vi "genIOL_realtime_traj.vi"() -> ()   [LabVIEW 2016]
panel:
  out "1-D Array of Real 2":dbl[](array[numeric])
  out "1-D Array of Real":dbl[](array[numeric])
  in  "Bscan path":path=path "D:/IRISSoft LV2016 beta/Host Demo/ThorlabsData/Incision Bscan/test.png"
  in  "size_xyz":dbl[](array[numeric])=[400.0, 400.0, 1024.0, 1.0]
  in  "size_xyz_mm":dbl[](array[numeric])=[16.0, 16.0, 9.4, 1.0]
  in  "incision row range":dbl=0.09
  in  "Incision point":dbl[](array[numeric])=[5.0, 9.897598828696928, 1.731822640236092]
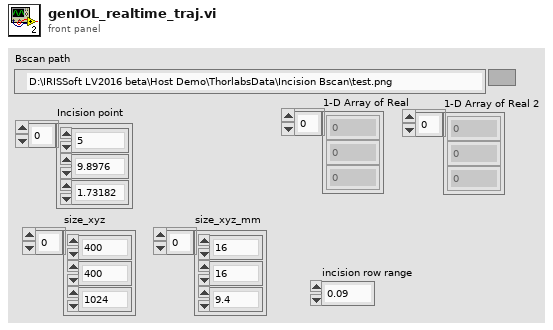
[diagram p1: front panel]
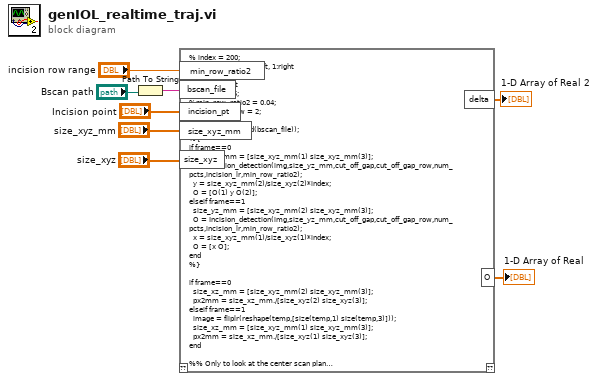
[diagram p0: block diagram]
diagram:
  n1 = Path To String(path="Bscan path") -> (string=w4:string)
  n2 = script code="% index = 200;\nincision_lr = 0; % 0:left, 1:right\ncut_off_gap = 3.5;\n% 0 < init_pct\nnum_pcts = 5;\n%min_row_ratio2 = 0.04;\ncut_off_gap_row = 2;\n\nimg = fliplr(imread(bscan_file));\n%{\nif frame==0\n  size_yz_mm = [size_xyz_mm(1) size_xyz_mm(3)];\n  O = Incision_detection(img,size_yz_mm,cut_off_gap,cut_off_gap_row,num_pcts,incision_lr,min_row_ratio2);\n  y = size_xyz_mm(2)/size_xyz(2)*index;\n  O = [O(1) y O(2)];\nelseif frame==1\n  size_yz_mm = [size_xyz_mm(2) size_xyz_mm(3)];\n  O = Incision_detection(img,size_yz_mm,cut_off_gap,cut_off_gap_row,num_pcts,incision_lr,min_row_ratio2);\n  x = size_xyz_mm(1)/size_xyz(1)*index;\n  O = [x O];\nend\n%}\n\nif frame==0\n  size_xz_mm = [size_xyz_mm(2) size_xyz_mm(3)];\n  px2mm = size_xz_mm./[size_xyz(2) size_xyz(3)]; \nelseif frame==1\n  image = fliplr(reshape(temp,[size(temp,1) size(temp,3)]));\n  size_xz_mm = [size_xyz_mm(1) size_xyz_mm(3)];\n  px2mm = size_xz_mm./[size_xyz(1) size_xyz(3)]; \nend\n\n%% Only to look at the center scan plan\nfigure(2); clf; \nimshow(img); hold on;\n    \n% Collect two user clicks of Injection location \n[input1, Zinput1] = ginput(1);\nplot(input1, Zinput1, 'rx', 'MarkerSize', 20, 'LineWidth', 3); \n[input2, Zinput2] = ginput(1); % Collect two user clicks \nplot(input2, Zinput2, 'rx', 'MarkerSize', 20, 'LineWidth', 3); \nif frame==1\n  Yinput1 = size_xyz(2) - input1; \n  Yinput2 = size_xyz(2) - input2;\nelseif frame==0\n  Yinput1 = size_xyz(1) - input1; \n  Yinput2 = size_xyz(1) - input2;\nend\n\nINJECTloc_px = [Yinput1, Zinput1; ... \n        Yinput2, Zinput2]; % [px] \nINJECTloc_px_mid=[(INJECTloc_px(1,1)+INJECTloc_px(2,1))/2,(INJECTloc_px(1,2)+INJECTloc_px(2,2))/2];\nclose(2); % close figure\n    \n% Convert these two locations from pixels to {OCT} frame  \nxloc_OCT = index/400*size_xz_mm(1); % B-scan is halfway through the image\nINJECTloc_OCT = [xloc_OCT*ones(1,1), INJECTloc_px_mid(1,1)*px2mm(1),  INJECTloc_px_mid(1,2)*px2mm(2)];\n%INJECTloc_OCT = [xloc_OCT*ones(1,1), INJECTloc_px_mid(1,1)*px2mm(1),  (INJECTloc_px_mid(1,2)*px2mm(2)-1.6)/4.8*9.4];\n\nif frame==0\n  O = [INJECTloc_OCT(2), INJECTloc_OCT(1), INJECTloc_OCT(3)];\nelse\n  O = INJECTloc_OCT(1:3);\nend\n\nTOI_file= 'D:\\IRISSoft LV2016 beta\\Host Demo\\TOI_static'\nfid_TOI = fopen(TOI_file,'r');\nTOI=fscanf(fid_TOI,'%f');\nTOI= reshape(TOI, [4 4])';\nfclose(fid_TOI);\n\nO(1) = O(1)-(size_xyz_mm(1)-10)/2;\nO(2) = O(2)-(size_xyz_mm(2)-10)/2;\nnew_incision_pt = inv(TOI)*[O(1);O(2);O(3);1];\n\nincision_pt = [incision_pt(1) incision_pt(2) incision_pt(3) 1]';\nO = inv(TOI)*incision_pt;\n\ndelta = new_incision_pt(1:3)-O(1:3);\ndelta = delta';\nO = O';\n% transformation\ndelta(2) = -delta(2);\ndelta(3) = -delta(3);"("min_row_ratio2"="incision row range", "bscan_file"=w4, "incision_pt"="Incision point", "size_xyz_mm"="size_xyz_mm", "size_xyz"="size_xyz") -> ("delta"=→"1-D Array of Real 2":dbl[], "O"=→"1-D Array of Real":dbl[])  [unwired: 1 in, 1 out]
